vi "Set_TDMSprops.vi"(8 "error in (no error)":errorcluster, 10 "Path":path, 11 "tdms file":refnum<k34>) -> (0 "error out":errorcluster, 3 "tdms file out":refnum<k34>)   [LabVIEW 2012]
uses:
  <vilib>/Utility/file.llb/Read From Spreadsheet File (string).vi
panel:
  out "all rows":string[][](array[string])
  out "propvals":string[][](array[string])
  out "channel names":string[](array[string])
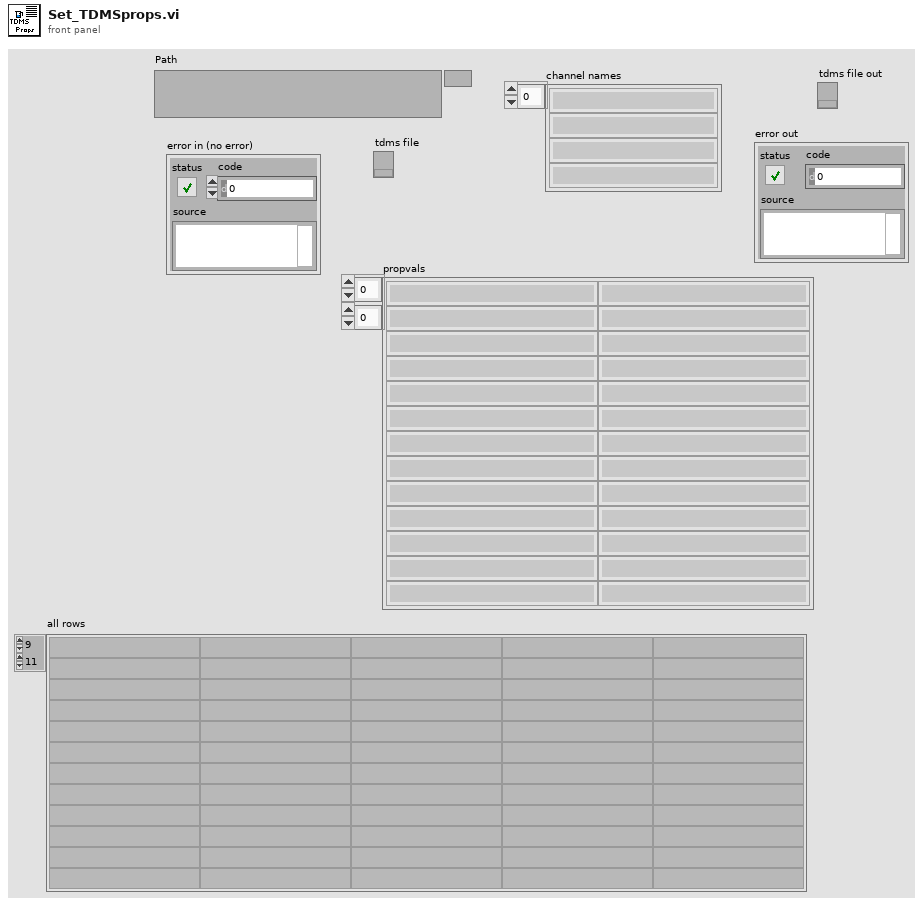
[diagram p1: front panel]
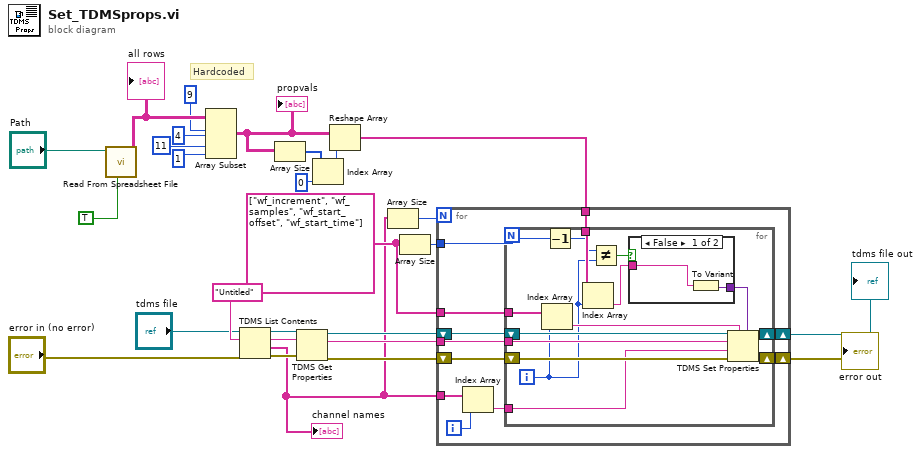
[diagram p0: block diagram]
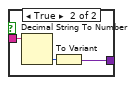
[diagram p2: hidden frame]
diagram:
  w5 = string[] ["wf_increment", "wf_samples", "wf_start_offset", "wf_start_time"] ("property names")
  # "Hardcoded"
  n1 = call-poly <vilib>:"Read From Spreadsheet File.vi"("transpose (no:F)"=TRUE, "file path (dialog if empty)"="Path") -> ("all rows"=w16:string[][])  [unwired: 5 in, 4 out]
  "all rows" <- w16
  n2 = Array Subset(array=w16, index (row)=9 ("index"), length (row)=4 ("length"), index (col)=11 ("index"), length (col)=1 ("length")) -> (w9:string[][])
  "propvals" <- w9
  n3 = TDMS List Contents(4:"error in (no error)", 6:"Untitled" ("group name"), 7:"tdms file") -> (0:w22:errorcluster, 1:w3:string[], 2:w20:string, 3:w23:refnum<k34>)
  "channel names" <- w3
  n4 = Array Size(array=w9) -> (size(s)=w10:i32[])
  n5 = TDMS Get Properties(8:w22, 10:w20, 11:w23) -> (0:w26:errorcluster, 2:w19:string, 3:w27:refnum<k34>)  [unwired: 3 in, 3 out]
  n6 = Index Array(array=w10, index=0) -> (element=w11:i32)
  n7 = Reshape Array(w9, w11) -> (w8:string[])
  n8 = Array Size(array=w3) -> (size(s)=w4:i32)
  n9 = Array Size(array=w5) -> (size(s)=w7:i32)
  n10 = for {
    N: w4 -> [_]
    tunnel: w19 -> [w34]
    tunnel: w8 -> [w33]
    tunnel: w7 -> [w32]
    tunnel: w5 -> [w31]
    shift-right: [w36] -> w25
    shift-left: w27 -> [w38]
    shift-right: [w35] -> w24
    shift-left: w26 -> [w37]
    tunnel: w3 -> [w30]
    i -> [w29]
    n11 = Index Array(array=w30, index=w29) -> (element=w28:string)
    n12 = for {
      N: w32 -> [w42]
      tunnel: w34 -> [w49]
      shift-right: [w51] -> w36
      shift-left: w38 -> [w53]
      shift-right: [w50] -> w35
      shift-left: w37 -> [w52]
      tunnel: w33 -> [w48]
      tunnel: w31 -> [w47]
      tunnel: w28 -> [w45]
      i -> [w43]
      n13 = Index Array(array=w47, index=w43) -> (element=w46:string)
      n14 = Decrement(x=w42) -> (x-1=w39:i32)
      n15 = Index Array(array=w48, index=w43) -> (element=w41:string)
      n16 = Not Equal?(x=w39, y=w43) -> (x != y?=w44:bool)
      n17 = case shown="False" w44 {
        tunnel: w41 -> [w54 w58]
        tunnel: [w55 w56] -> w40
        frame False {
          n18 = To Variant(anything=w54) -> (Variant=w55:variant)
        }
        frame True {
          n19 = Decimal String To Number(string=w58) -> (number=w57:i32)  [unwired: 2 in, 1 out]
          n20 = To Variant(anything=w57) -> (Variant=w56:variant)
        }
      }
      n21 = TDMS Set Properties(5:w40, 7:w46, 8:w52, 9:w45, 10:w49, 11:w53) -> (0:w50:errorcluster, 3:w51:refnum<k34>)  [unwired: 2 out]
    }
  }
  "tdms file out" <- w25
  "error out" <- w24
